vi "SubVI_AdvancedHowdyDrive_TeleOp.vi"(5 "Max Acceleration\n(native units)":dbl=72000.0 format="%#_13g", 7 "Max Output\n(native units)":dbl=38000.0 format="%#_13g", 8 "error in (no error)":errorcluster, 9 "Y axis value":dbl, 10 "X axis value":dbl, 11 "RobotDriveDevRef":T1={"DevStatus"={"status"=FALSE, "code"=0, "source"=""}, "Motors[]"=[], "Square Inputs"=FALSE, "Max Output"=1.0}) -> (0 "error out":errorcluster, 3 "RobotDriveDevRef 2":T1={"DevStatus"={"status"=FALSE, "code"=0, "source"=""}, "Motors[]"=[], "Square Inputs"=FALSE, "Max Output"=1.0})   [LabVIEW 2017]
uses:
  <vilib>/Rock Robotics/WPI/RobotDrive/WPI_RobotDriveDevRef.ctl
  <vilib>/Rock Robotics/WPI/MotorControl/WPI_MotorControlDeviceRef.ctl
  <vilib>/Rock Robotics/WPI/MotorControl/WPI_MotorControlType.ctl
  <vilib>/Rock Robotics/SystemInterfaces/DIO/FPGA_DIOPWMChannel.ctl
  <vilib>/Rock Robotics/WPI/PWM/WPI_PWMDeadband.ctl
  <vilib>/Rock Robotics/SystemInterfaces/DIO/FPGA_DIOChannel.ctl
  <vilib>/Rock Robotics/SystemInterfaces/NetworkCommunication/NetComm_UsageReport_ResourceType.ctl
panel:
  in  "turn rate":dbl=30000.0 format="%#_13g"
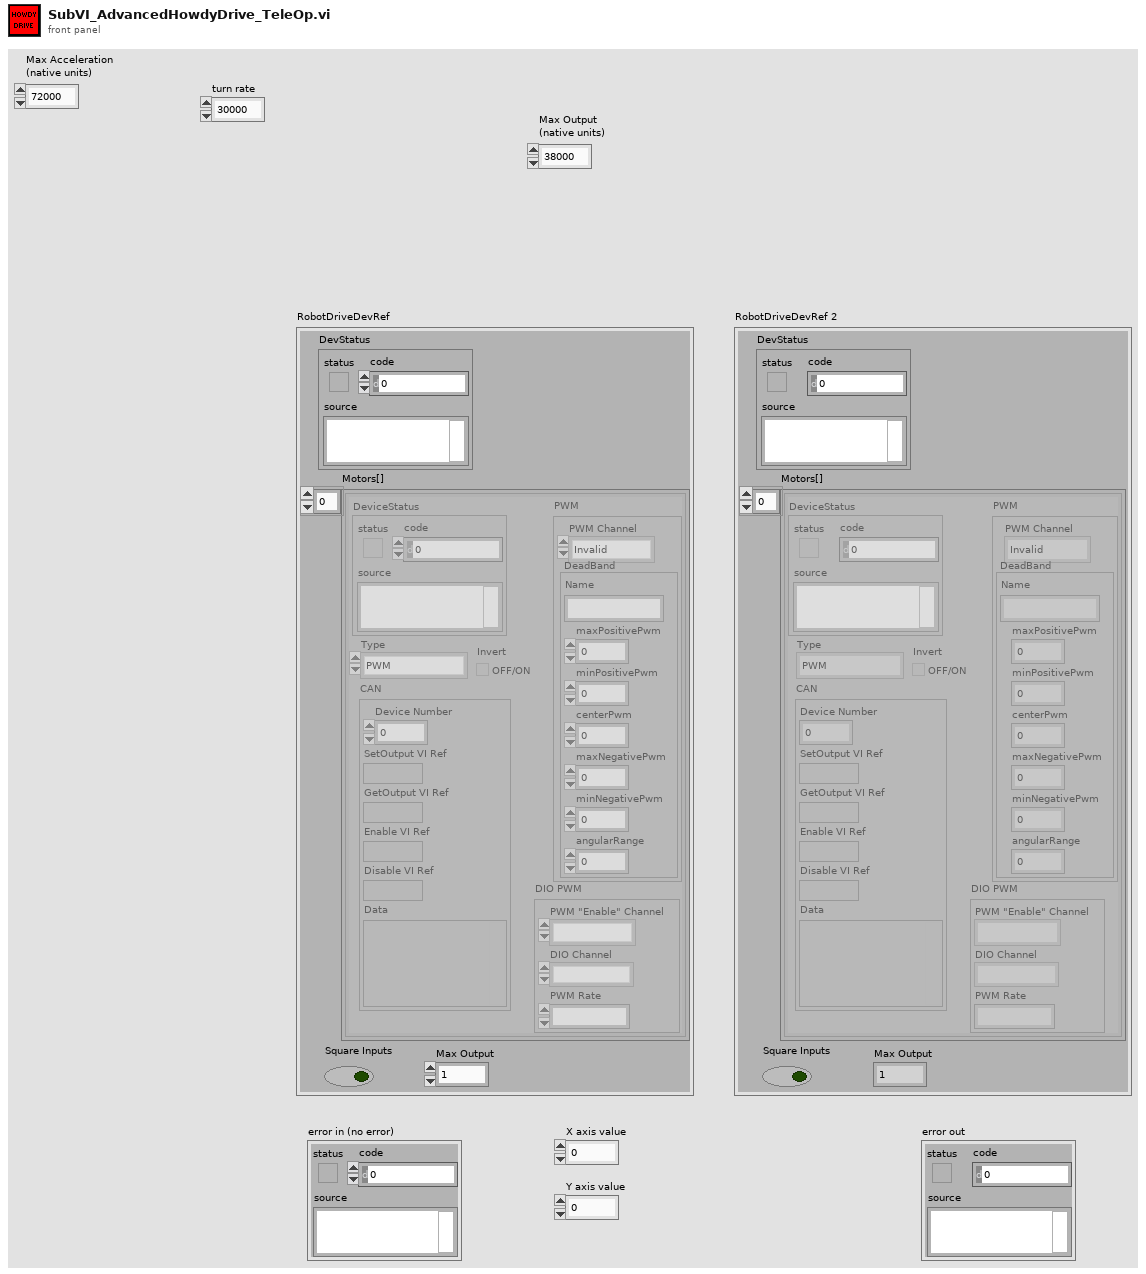
[diagram p1: front panel]
types:
  T1 = typedef "WPI_RobotDriveDevRef.ctl" = cluster{"DevStatus":errorcluster, "Motors[]":T2[], "Square Inputs":bool, "Max Output":dbl}
  T2 = typedef "WPI_MotorControlDeviceRef.ctl" = cluster{"DeviceStatus":errorcluster, "Type":T3, "PWM":cluster{"PWM Channel":T4, "DeadBand":T5}, "CAN":cluster{"Device Number":u8, "SetOutput VI Ref":variant, "GetOutput VI Ref":variant, "Enable VI Ref":variant, "Disable VI Ref":variant, "Data":variant}, "Invert":bool, "DIO PWM":cluster{"PWM \"Enable\" Channel":T4, "DIOChannel":T6, "PWM Rate":dbl}}
  T3 = typedef "WPI_MotorControlType.ctl" = enum16{"PWM", "CAN", "DIO PWM"}
  T4 = typedef "FPGA_DIOPWMChannel.ctl" = enum8{"PWM 0", "PWM 1", "PWM 2", "PWM 3", "PWM 4", "PWM 5", "PWM 6", "PWM 7", "PWM 8", "PWM 9", "PWM MXP 0", "PWM MXP 1", "PWM MXP 2", "PWM MXP 3", "PWM MXP 4", "PWM MXP 5", "PWM MXP 6", "PWM MXP 7", "PWM MXP 8", "PWM MXP 9", "Invalid"}
  T5 = typedef "WPI_PWMDeadband.ctl" = cluster{"Name":string, "maxPositivePwm":i32, "minPositivePwm":i32, "centerPwm":i32, "maxNegativePwm":i32, "minNegativePwm":i32, "angularRange":u16}
  T6 = typedef "FPGA_DIOChannel.ctl" = enum8{"DIO 0", "DIO 1", "DIO 2", "DIO 3", "DIO 4", "DIO 5", "DIO 6", "DIO 7", "DIO 8", "DIO 9", "DIO MXP 0", "DIO MXP 1", "DIO MXP 2", "DIO MXP 3", "DIO MXP 4", "DIO MXP 5", "DIO MXP 6", "DIO MXP 7", "DIO MXP 8", "DIO MXP 9", "DIO MXP 10", "DIO MXP 11", "DIO MXP 12", "DIO MXP 13", "DIO MXP 14", "DIO MXP 15", "SPI Port CS1", "SPI Port CS2", "SPI Port CS3", "SPI Port MISO", "SPI Port MOSI", "Invalid"}
  T7 = typedef "NetComm_UsageReport_ResourceType.ctl" = enum8{"Controller", "Module", "Language", "CANPlugin", "Accelerometer", "ADXL345", "AnalogChannel", "AnalogTrigger", "AnalogTriggerOutput", "CANJaguar", "Compressor", "Counter", "Dashboard", "DigitalInput", "DigitalOutput", "DriverStationCIO", "DriverStationEIO", "DriverStationLCD", "Encoder", "GearTooth", "Gyro", "I2C", "Framework", "Jaguar", "Joystick", "Kinect", "KinectStick", "PIDController", "Preferences", "PWM", "Relay", "RobotDrive", "SerialPort", "Servo", "Solenoid", "SPI", "Task", "Ultrasonic", "Victor", "Button", "Command", "AxisCamera", "PCVideoServer", "SmartDashboard", "Talon", "HiTechnicColorSensor", "HiTechnicAccel", "HiTechnicCompass", "SRF08", "AnalogOutput", "Victor SP", "Talon SRX", "CAN Talon SRX", "ADXL362 Accel", "ADXRS450 Gyro", "Rev SPARK", "Mindsensors SD540", "Digital Filter", "ADIS16448", "PDP", "PCM", "PigeonIMU", "Nidec Brushless", "CTRE CANifier", "CTRE Future 0", "CTRE Future 1", "CTRE Future 2", "CTRE Future 3", "CTRE Future 4", "CTRE Future 5", "CTRE Future 6"}
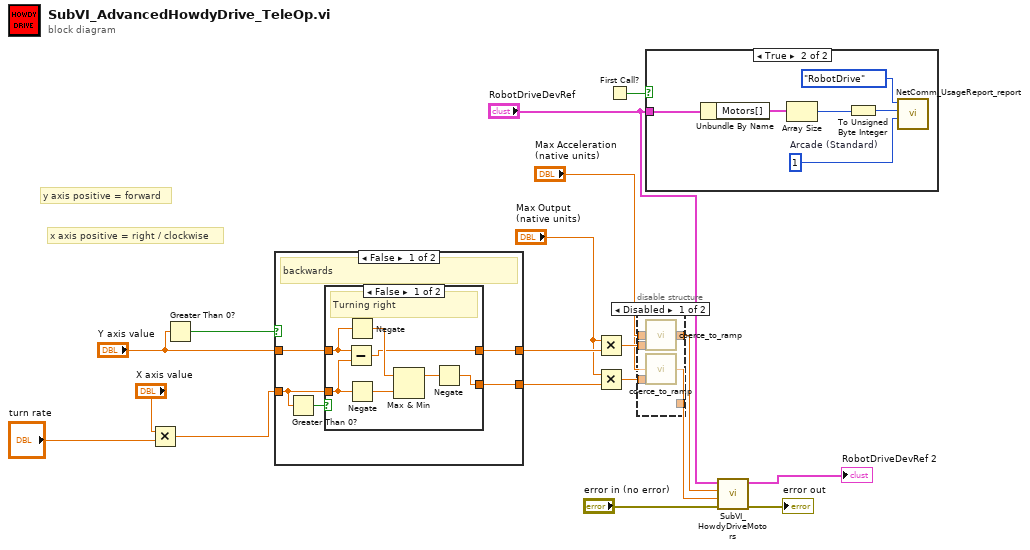
[diagram p0: block diagram]
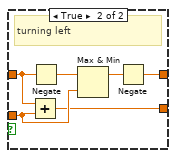
[diagram p3: hidden frame]
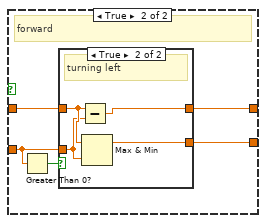
[diagram p4: hidden frame]
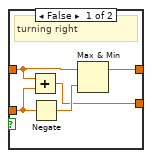
[diagram p5: hidden frame]
diagram:
  # "x axis positive = right / clockwise"
  # "y axis positive = forward"
  n1 = Multiply(x="X axis value", y="turn rate") -> (x*y=w1:dbl)
  n2 = Greater Than 0?(x="Y axis value") -> (x > 0?=w6:bool)
  n3 = case shown="False" w6 {
    tunnel: w1 -> [w22 w40]
    tunnel: "Y axis value" -> [w21 w39]
    tunnel: [w20 w38] -> w7
    tunnel: [w19 w37] -> w8
    frame False {
      # "backwards"
      n4 = Greater Than 0?(x=w22) -> (x > 0?=w23:bool)
      n5 = case shown="False" w23 {
        tunnel: w22 -> [w30 w32]
        tunnel: w21 -> [w28 w33]
        tunnel: [w24 w34] -> w20
        tunnel: [w25 w31] -> w19
        frame False {
          # "Turning right"
          n6 = Subtract(x=w28, y=w30) -> (x-y=w24:dbl)
          n7 = Negate(x=w28) -> (-x=w29:dbl)
          n8 = Negate(x=w30) -> (-x=w27:dbl)
          n9 = Max & Min(x=w29, y=w27) -> (max(x,y)=w26:dbl)  [unwired: 1 out]
          n10 = Negate(x=w26) -> (-x=w25:dbl)
        }
        frame True {
          # "turning left"
          n11 = Add(x=w33, y=w32) -> (x+y=w31:dbl)
          n12 = Negate(x=w33) -> (-x=w36:dbl)
          n13 = Max & Min(x=w36, y=w32) -> (max(x,y)=w35:dbl)  [unwired: 1 out]
          n14 = Negate(x=w35) -> (-x=w34:dbl)
        }
      }
    }
    frame True {
      # "forward"
      n15 = Greater Than 0?(x=w40) -> (x > 0?=w41:bool)
      n16 = case shown="True" w41 {
        tunnel: w40 -> [w46 w48]
        tunnel: w39 -> [w43 w49]
        tunnel: [w44 w47] -> w38
        tunnel: [w42 w50] -> w37
        frame False {
          # "turning right"
          n17 = Add(x=w43, y=w46) -> (x+y=w42:dbl)
          n18 = Negate(x=w46) -> (-x=w45:dbl)
          n19 = Max & Min(x=w43, y=w45) -> (max(x,y)=w44:dbl)  [unwired: 1 out]
        }
        frame True {
          # "turning left"
          n20 = Subtract(x=w49, y=w48) -> (x-y=w47:dbl)
          n21 = Max & Min(x=w49, y=w48) -> (max(x,y)=w50:dbl)  [unwired: 1 out]
        }
      }
    }
  }
  n22 = Multiply(x="Max Output\n(native units)", y=w7) -> (x*y=w12:dbl)
  n23 = Multiply(x="Max Output\n(native units)", y=w8) -> (x*y=w10:dbl)
  n24 = First Call?() -> (First Call?: T/F=w18:bool)
  n25 = disable-structure shown="Disabled" {
    disable-tunnel: "Max Acceleration\n(native units)" -> [w55 _]
    disable-tunnel: w12 -> [w54 w57]
    disable-tunnel: [w53 w57] -> w11
    disable-tunnel: w10 -> [w52 w56]
    disable-tunnel: [w51 w56] -> w9
    frame Disabled {
      n26 = call "coerce_to_ramp.vi"("Requested speed\n(native units)"=w54, "Max Acceleration\n(native units)/second"=w55) -> ("Ramped speed\n(percent)"=w53:dbl)  [unwired: 1 in]
      n27 = call "coerce_to_ramp.vi"("Requested speed\n(native units)"=w52, "Max Acceleration\n(native units)/second"=w55) -> ("Ramped speed\n(percent)"=w51:dbl)  [unwired: 1 in]
    }
    frame Enabled {
    }
  }
  n28 = case shown="True" w18 {
    tunnel: "RobotDriveDevRef" -> [_ w59]
    frame False {
    }
    frame True {
      w61 = u8 1  # Arcade (Standard)
      n29 = Unbundle By Name(w59) -> ("Motors[]"=w58:T2[])
      n30 = Array Size(array=w58) -> (size(s)=w60:i32)
      n31 = To Unsigned Byte Integer(number=w60) -> (unsigned 8bit integer=w62:u8)
      n32 = call <vilib>:"NetComm_UsageReport_report.vi"("Context"=w61, "Instance Number"=w62, "Resource Type"=NetComm_UsageReport_ResourceType."RobotDrive") -> ()  [unwired: 9 in]
    }
  }
  n33 = call "SubVI_HowdyDriveMotors.vi"("error in (no error)"="error in (no error)", "RightSpeed"=w9, "LeftSpeed"=w11, "RobotDriveDevRef 2"="RobotDriveDevRef") -> ("error out"=→"error out":errorcluster, "RobotDriveDevRef"=→"RobotDriveDevRef 2":T1)  [unwired: 6 in]
